vi "ReadWrite.ProcessData.Read.vi"(7 "Ignore Reset Values?":bool=TRUE, 8 "error in":errorcluster, 10 "timeout ms":i32=100, 11 "ReadWrite in":refnum<class "ReadWrite.lvclass">) -> (0 "error out":errorcluster, 1 "Timeout?":bool, 2 "Values":dbl[](array[numeric]), 3 "ReadWrite out":refnum<class "ReadWrite.lvclass">, 5 "Detect?":bool[](array[boolean]))   [LabVIEW 2024, in "VS Plugin Data Access Engine.lvlib" / "ReadWrite.lvclass"]
uses:
  ReadWrite.lvclass
  ReadWrite.lvclass/ReadWrite.ctl
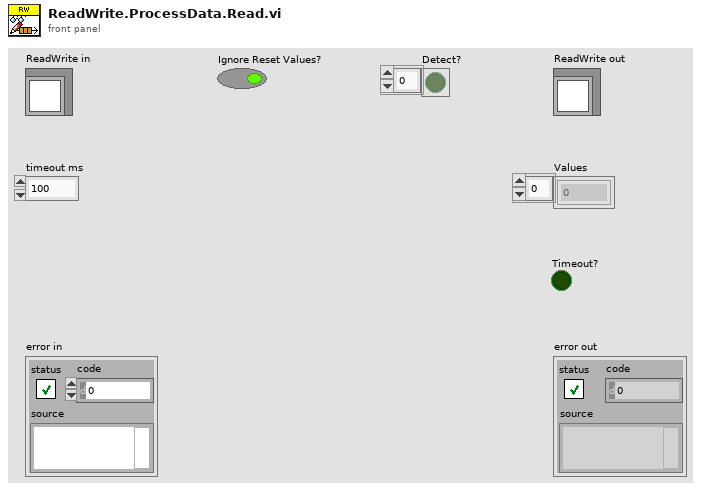
[diagram p1: front panel]
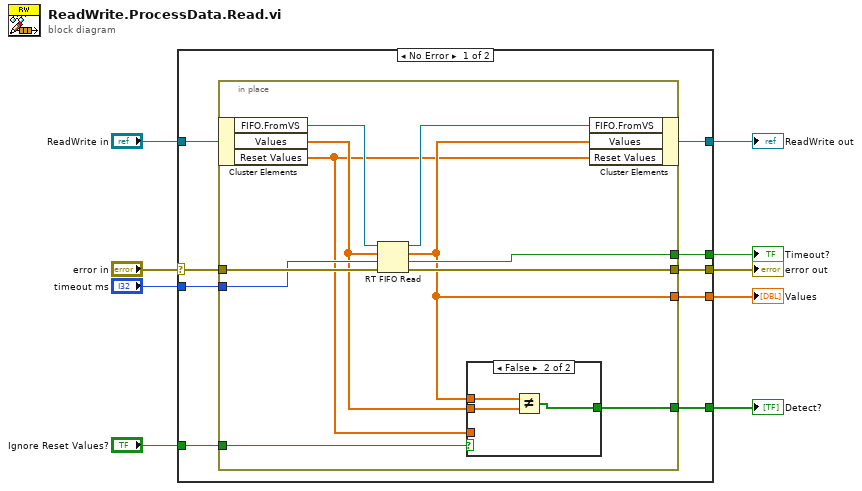
[diagram p0: block diagram]
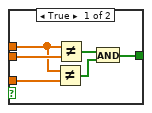
[diagram p2: hidden frame]
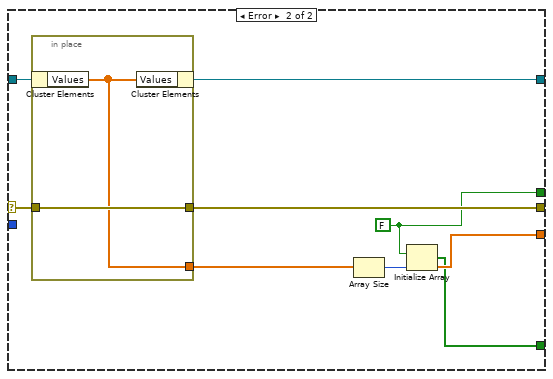
[diagram p3: hidden frame]
diagram:
  n1 = case shown="No Error" "error in" {
    selector: "error in" -> [w18 w45]
    tunnel: [w17 w46] -> w8
    tunnel: [w14 w43] -> w2
    tunnel: "ReadWrite in" -> [w15 w44]
    tunnel: [w16 w41] -> w7
    tunnel: "timeout ms" -> [w13 _]
    tunnel: [w12 w39] -> w5
    tunnel: [w11 w40] -> w4
    tunnel: "Ignore Reset Values?" -> [w10 _]
    frame No Error {
      n2 = in-place {
        in-place-border: w18 -> [w29]
        in-place-border: [w28] -> w17
        in-place-border: [w21] -> w16
        in-place-border: w13 -> [w25]
        in-place-border: [w24] -> w12
        in-place-border: [w22] -> w11
        in-place-border: w10 -> [w20]
        n3 = in-place-cluster #1(w15) -> ("FIFO.FromVS"=w27:refnum<k33>, "Values"=w23:dbl[], "Reset Values"=w19:dbl[])
        n4 = RT FIFO Read(0:w27, 1:w23, 2:w25, 3:w29) -> (8:w26:refnum<k33>, 9:w21:dbl[], 10:w24:bool, 11:w28:errorcluster)  [unwired: 1 out]
        n5 = case shown="False" w20 {
          tunnel: w23 -> [w35 w38]
          tunnel: [w31 w36] -> w22
          tunnel: w21 -> [w33 w37]
          tunnel: w19 -> [w32 _]
          frame True {
            n6 = Not Equal?(x=w33, y=w32) -> (x != y?=w30:bool[])
            n7 = Not Equal?(x=w33, y=w35) -> (x != y?=w34:bool[])
            n8 = And(x=w34, y=w30) -> (x .and. y?=w31:bool[])
          }
          frame False {
            n9 = Not Equal?(x=w37, y=w38) -> (x != y?=w36:bool[])
          }
        }
        n10 = in-place-cluster #1("FIFO.FromVS"=w26, "Values"=w21, "Reset Values"=w19) -> (w14:refnum<class "ReadWrite.lvclass">)
      }
    }
    frame Error {
      w39 = FALSE ("empty?")
      n11 = in-place {
        in-place-border: [w47] -> w41
        in-place-border: [w48] -> w46
        in-place-border: w45 -> [w48]
        n12 = in-place-cluster #2(w44) -> ("Values"=w47:dbl[])
        n13 = in-place-cluster #2("Values"=w47) -> (w43:refnum<class "ReadWrite.lvclass">)
      }
      n14 = Array Size(array=w41) -> (size(s)=w42:i32)
      n15 = Initialize Array(w39, w42) -> (w40:bool[])
    }
  }
  "error out" <- w8
  "ReadWrite out" <- w2
  "Values" <- w7
  "Timeout?" <- w5
  "Detect?" <- w4
